vi "Height_fb (SubVI).vi"(6 "Height_pcc":dbl, 7 "height_set_point":dbl, 9 "height_pg":dbl, 10 "step_upper_lim":dbl, 11 "step_lower_lim":dbl) -> (2 "hieght_fb_out":dbl, 3 "height_fb":dbl)   [LabVIEW 2022 SP3]
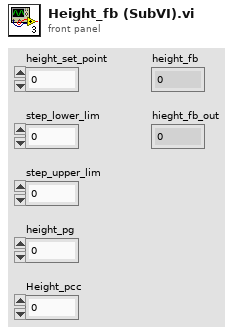
[diagram p1: front panel]
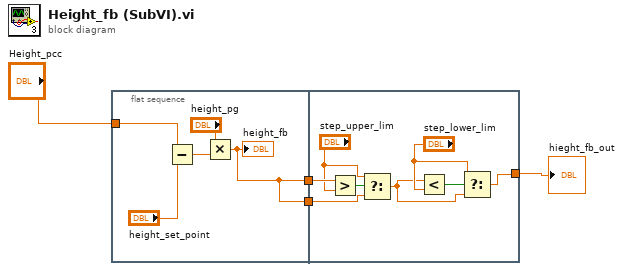
[diagram p0: block diagram]
diagram:
  n1 = flat-sequence {
    tunnel: "Height_pcc" -> [w9]
    tunnel: [w5] -> w4
    tunnel: [w5] -> w3
    tunnel: w4 -> [w17]
    tunnel: w3 -> [w14]
    tunnel: [w10] -> w2
    frame #0 {
      n2 = Subtract(x=w9, y="height_set_point") -> (x-y=w7:dbl)
      n3 = Multiply(x="height_pg", y=w7) -> (x*y=w5:dbl)
      "height_fb" <- w5
    }
    frame #1 {
      n4 = Greater?(x=w17, y="step_upper_lim") -> (0:w16:bool)
      n5 = Select(t="step_upper_lim", s=w16, f=w14) -> (s? t:f=w11:dbl)
      n6 = Less?(x=w11, y="step_lower_lim") -> (x < y?=w12:bool)
      n7 = Select(t="step_lower_lim", s=w12, f=w11) -> (s? t:f=w10:dbl)
    }
  }
  "hieght_fb_out" <- w2
